vi "EmergencyPT (1).vi"(1 "Numeric":dbl) -> (0 "Boolean":bool)   [LabVIEW 2017]
uses:
  EmergencyGLOBAL.vi
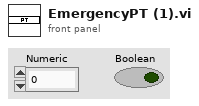
[diagram p1: front panel]
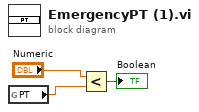
[diagram p0: block diagram]
diagram:
  n1 = global read "EmergencyGLOBAL.vi" "PT"() -> (w1:dbl)
  n2 = Less?(x="Numeric", y=w1) -> (x < y?=→"Boolean":bool)
